vi "Ejercicio 4.3.vi"() -> ()   [LabVIEW 2021]
panel:
  out "Número de 1":i16
  out "Número de 0":i16
  out "Waveform Chart":i16[](graph)
  in  "stop":bool
  out "data":bool[](array[boolean])
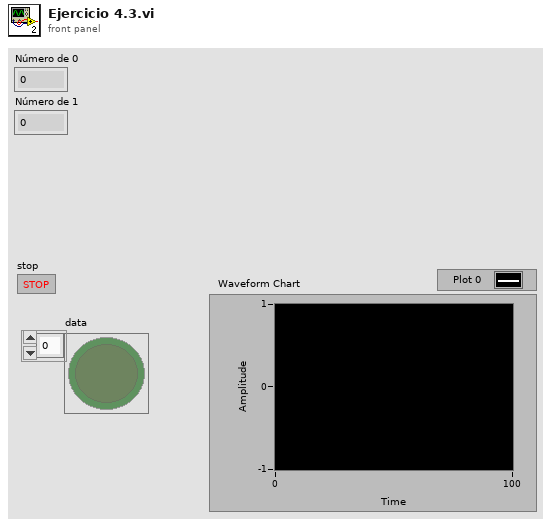
[diagram p1: front panel]
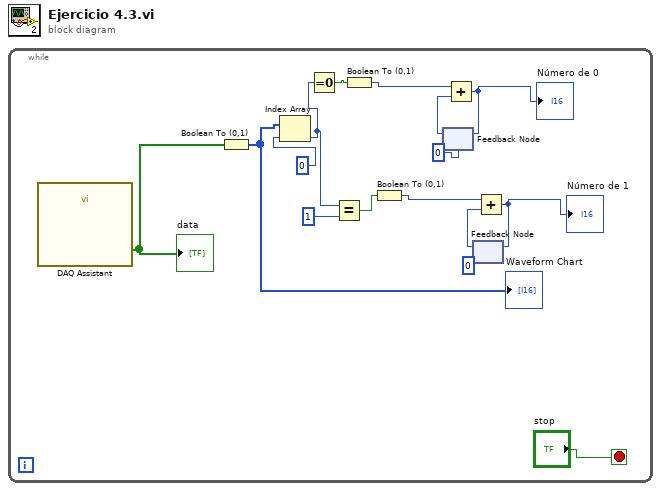
[diagram p0: block diagram]
diagram:
  n1 = while {
    stop <- "stop" stop-if-true
    (unwired) 0
    n2 = call "DAQ Assistant"() -> ("data"=w14:bool[])  [unwired: 17 in, 2 out]
    "data" <- w14
    n3 = Boolean To (0,1)(Boolean=w14) -> (0, 1=w8:i16[])
    "Waveform Chart" <- w8
    n4 = Index Array(array=w8, index=0) -> (element=w5:i16)
    n5 = Equal To 0?(x=w5) -> (x = 0?=w11:bool)
    n6 = Equal?(x=w5, y=1) -> (x = y?=w1:bool)
    n7 = Boolean To (0,1)(Boolean=w11) -> (0, 1=w12:i16)
    n8 = Boolean To (0,1)(Boolean=w1) -> (0, 1=w3:i16)
    n9 = feedback #1(0) -> (w13:i32)
    n10 = Add(x=w12, y=w13) -> (x+y=w9:i32)
    "Número de 0" <- w9
    n11 = feedback-in #1(w9) -> ()
    n12 = feedback #2() -> (w4:i16)  [unwired: 1 in]
    n13 = Add(x=w3, y=w4) -> (x+y=w2:i16)
    "Número de 1" <- w2
    n14 = feedback-in #2(w2) -> ()
  }
